vi "Fsweep_SR8XX.vi"() -> ()   [LabVIEW 2025]
panel:
  out "Array":dbl[](array[numeric])=[40.99999999999999, 50.30821597193005, 61.72967303117947, 75.74413957876105, 92.94030567161772, 114.04051146890099, 139.93108976894726, 171.6995972020422, 210.68049800813995, 258.511219387007, 317.2009330753302, 389.2149523817426, 477.57828985183363, 586.0027255944161, 719.042723886428, 882.2867474712998, 1082.5920058770212, 1328.3724985645404, 1629.9524524135916, 2000.0000000000002]
  in  "data acq time (s)":dbl=2.0
  in  "restart":bool
  in  "stop":bool
  in  "coupled device":enum16{"SRS 8XXX", "Keithley 6221"}(ring)
  in  "base delay (ms)":dbl=2000.0
  in  "test mode":bool
  out "done":u32=1
  out "delays (ms)":dbl[](array[numeric])=[4439.024390243903, 3987.7468931873063, 3619.966461664074, 3320.2341535085625, 3075.9594481357317, 2876.881370593205, 4439.024390243903, 3987.7468931873063, 3619.966461664074, 3320.2341535085625, 3075.9594481357317, 2876.881370593205, 2714.6374702370927, 4439.024390243903, 3987.7468931873063, 3619.966461664074, 3320.2341535085625, 3075.9594481357317, 2876.881370593205, 2714.6374702370927]
  in  "back to initial frequencies":bool=TRUE
  out "delay sum (min)":dbl=1.823145218207876
  in  "index offset":u16=150
  out "freq profile":dbl[][](array[numeric])=[[40.99999999999999, 171.6995972020422, 719.042723886428], [50.30821597193005, 210.68049800813995, 882.2867474712998], [61.72967303117947, 258.511219387007, 1082.5920058770212], [75.74413957876105, 317.2009330753302, 1328.3724985645404], [92.94030567161772, 389.2149523817426, 1629.9524524135916], [114.04051146890099, 477.57828985183363, 2000.0000000000002], [139.93108976894726, 586.0027255944161, 40.99999999999999], [171.6995972020422, 719.042723886428, 50.30821597193005], [210.68049800813995, 882.2867474712998, 61.72967303117947], [258.511219387007, 1082.5920058770212, 75.74413957876105], [317.2009330753302, 1328.3724985645404, 92.94030567161772], [389.2149523817426, 1629.9524524135916, 114.04051146890099], [477.57828985183363, 2000.0000000000002, 139.93108976894726], [586.0027255944161, 40.99999999999999, 171.6995972020422], [719.042723886428, 50.30821597193005, 210.68049800813995], [882.2867474712998, 61.72967303117947, 258.511219387007], [1082.5920058770212, 75.74413957876105, 317.2009330753302], [1328.3724985645404, 92.94030567161772, 389.2149523817426], [1629.9524524135916, 114.04051146890099, 477.57828985183363], [2000.0000000000002, 139.93108976894726, 586.0027255944161]]
  out "freqs":dbl[](array[numeric])=[40.99999999999999, 171.6995972020422, 719.042723886428]
  out "delay (ms)":dbl=2714.6374702370927
  out "elapsed time (min)":dbl=2.0671833333333334
  in  "sweep mode":T1(ring)=enum."log"
  in  "size":u32=200
  in  "final":dbl=2000.0
  in  "initial":dbl=41.0
  in  "Device address":refnum<visa-resource-name>[](array[refnum])=["GPIB0::1::INSTR", "GPIB0::4::INSTR", "GPIB0::7::INSTR"]
  # "Test the frequency profile and the estimated measurement time (delay sum (min)) with the 'test mode on'\nTurn the test mode off for the real measurement."
  # "Start data acquistion and frequency sweeps.\nStop the data acqusition when the sweep is done.\nRepeat when 'restart' switch is ON.\nVISA resource is reused."
  # "this delay time is added to the frequency dependent delay time"
  # "(1) For multiple lockins, the same freq profile is used but\nbut the starting frequency is offset to prevent crosstalking.\n(2) Ignored for a single lockin. \n* Check the context help"
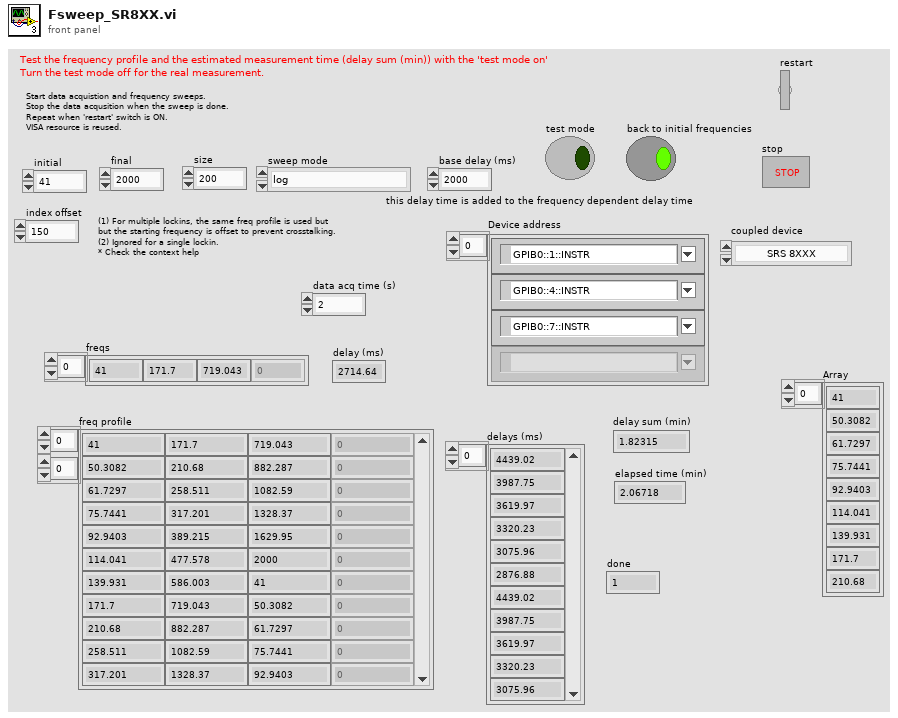
[diagram p1: front panel]
types:
  T1 = enum16{"linear", "inverse", "log", "inverse log"}
  T2 = enum32{"New", "Stop", "Trigger", "Delta Trigger", "Run", "Pause", "comments", "Started?"}
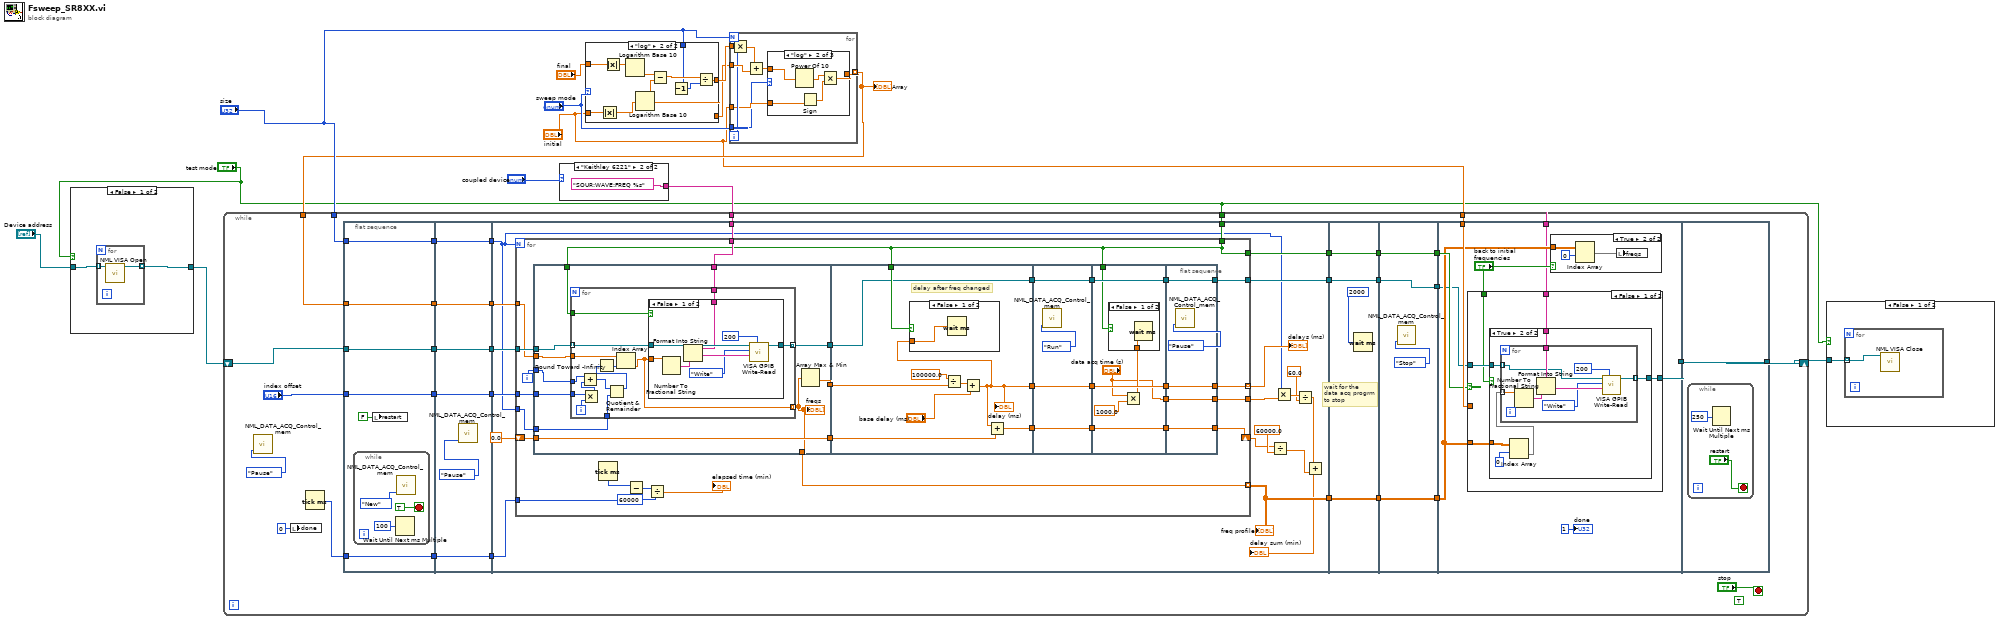
[diagram p0: block diagram]
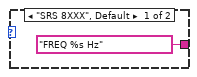
[diagram p10: hidden frame]
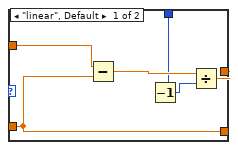
[diagram p11: hidden frame]
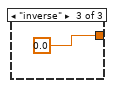
[diagram p13: hidden frame]
diagram:
  n1 = case shown="False" "test mode" {
    tunnel: [w15 w18] -> w4
    tunnel: "Device address" -> [w14 w18]
    frame False {
      n2 = for {
        tunnel: w14 -> [w17] mode=indexing
        tunnel: [w16] -> w15 mode=indexing
        n3 = call "NML VISA Open.vi"("VISA resource name"=w17) -> ("VISA resource name out"=w16:refnum<visa-resource-name>)  [unwired: 9 in, 1 out]
      }
    }
    frame True {
    }
  }
  n4 = case shown="\"Keithley 6221\"" "coupled device" {
    tunnel: ["FREQ %s Hz" ("format string") "SOUR:WAVE:FREQ %s" ("format string")] -> w5
    frame "SRS 8XXX", Default {
    }
    frame "Keithley 6221" {
    }
  }
  n5 = case shown="\"log\"" "sweep mode" {
    tunnel: "final" -> [w26 w27]
    tunnel: "initial" -> [w21 w32]
    tunnel: "size" -> [w24 w35]
    tunnel: [w23 w34] -> w13
    tunnel: [w21 w28] -> w12
    frame "linear", Default {
      n6 = Subtract(x=w26, y=w21) -> (x-y=w25:dbl)
      n7 = Decrement(x=w24) -> (x-1=w22:u32)
      n8 = Divide(x=w25, y=w22) -> (x/y=w23:dbl)
    }
    frame "log" {
      n9 = Absolute Value(x=w32) -> (abs(x)=w29:dbl)
      n10 = Absolute Value(x=w27) -> (abs(x)=w30:dbl)
      n11 = Logarithm Base 10(1:w30) -> (0:w31:dbl)
      n12 = Logarithm Base 10(1:w29) -> (0:w28:dbl)
      n13 = Subtract(x=w31, y=w28) -> (x-y=w36:dbl)
      n14 = Decrement(x=w35) -> (x-1=w33:u32)
      n15 = Divide(x=w36, y=w33) -> (x/y=w34:dbl)
    }
  }
  n16 = for {
    N: "size" -> [_]
    tunnel: w13 -> [w42]
    tunnel: [w44] -> w8 mode=indexing
    tunnel: "sweep mode" -> [w37]
    tunnel: w12 -> [w40]
    tunnel: "initial" -> [w38]
    i -> [w39]
    n17 = Multiply(x=w42, y=w39) -> (x*y=w41:dbl)
    n18 = Add(x=w41, y=w40) -> (x+y=w43:dbl)
    n19 = case shown="\"log\"" w37 {
      tunnel: [w45 w48 0.0] -> w44
      tunnel: w43 -> [w45 w50 _]
      tunnel: w38 -> [_ w47 _]
      frame "linear", Default {
      }
      frame "log" {
        n20 = Power Of 10(x=w50) -> (10^x=w49:dbl)
        n21 = Sign(1:w47) -> (0:w46:dbl)
        n22 = Multiply(x=w49, y=w46) -> (x*y=w48:dbl)
      }
      frame "inverse" {
      }
    }
  }
  "Array" <- w8
  n23 = while {
    tunnel: "size" -> [w55]
    tunnel: w8 -> [w61]
    tunnel: "initial" -> [w60]
    tunnel: w5 -> [w59]
    shift-right: [w57] -> w3
    shift-left: w4 -> [w58]
    tunnel: "test mode" -> [w53]
    stop <- "stop" stop-if-true
    (unwired) TRUE
    n24 = call "NML_DATA_ACQ_Control_mem.vi"("Enum"=T2."Pause") -> ()  [unwired: 5 in, 1 out]
    n25 = local write "done"(u32 0 ("done")) -> ()
    n26 = Tick Count (ms)() -> (millisecond timer value=w64:u32)
    n27 = flat-sequence {
      tunnel: "index offset" -> [w85]
      tunnel: w58 -> [w86]
      tunnel: w55 -> [w87]
      tunnel: w64 -> [w88]
      tunnel: w61 -> [w89]
      tunnel: [w89] -> w83
      tunnel: [w88] -> w82
      tunnel: [w87] -> w81
      tunnel: [w86] -> w80
      tunnel: [w85] -> w79
      tunnel: w83 -> [w98]
      tunnel: [w98] -> w78
      tunnel: w82 -> [w97]
      tunnel: [w97] -> w77
      tunnel: w81 -> [w96]
      tunnel: [w96] -> w76
      tunnel: w80 -> [w95]
      tunnel: [w95] -> w75
      tunnel: w79 -> [w94]
      tunnel: [w94] -> w74
      tunnel: [w117] -> w73
      tunnel: [w110] -> w72
      tunnel: w59 -> [w108]
      tunnel: [w107] -> w71
      tunnel: w78 -> [w118]
      tunnel: w77 -> [w116]
      tunnel: w76 -> [w104]
      tunnel: w75 -> [w111]
      tunnel: w74 -> [w115]
      tunnel: w53 -> [w106]
      tunnel: w73 -> [w214]
      tunnel: [w214] -> w70
      tunnel: w72 -> [w213]
      tunnel: [w213] -> w69
      tunnel: w71 -> [w212]
      tunnel: [w212] -> w68
      tunnel: w70 -> [w218]
      tunnel: [w218] -> w67
      tunnel: w69 -> [w217]
      tunnel: [w217] -> w66
      tunnel: [w216] -> w65
      tunnel: w68 -> [w216]
      tunnel: w67 -> [w225]
      tunnel: w60 -> [w226]
      tunnel: w66 -> [w222]
      tunnel: w59 -> [w221]
      tunnel: w65 -> [w219]
      tunnel: [w220] -> w54
      tunnel: [w251] -> w57
      tunnel: w54 -> [w251]
      frame #0 {
        n28 = while {
          stop <- TRUE stop-if-true
          n29 = Wait Until Next ms Multiple(millisecond multiple=u32 100) -> ()  [unwired: 1 out]
          n30 = call "NML_DATA_ACQ_Control_mem.vi"("Enum"=T2."New") -> ()  [unwired: 5 in, 1 out]
        }
        n31 = local write "restart"(FALSE ("restart")) -> ()
      }
      frame #1 {
        n32 = call "NML_DATA_ACQ_Control_mem.vi"("Enum"=T2."Pause") -> ()  [unwired: 5 in, 1 out]
      }
      frame #2 {
        n33 = for {
          N: w104 -> [_]
          tunnel: w118 -> [w135]
          tunnel: [w120] -> w117
          tunnel: w116 -> [w148]
          tunnel: w111 -> [w144]
          tunnel: w115 -> [w142]
          tunnel: w104 -> [w141]
          tunnel: [w136] -> w110 mode=indexing
          tunnel: [w119] -> w109 mode=indexing
          shift-right: [w139] -> w112
          shift-left: 0.0 -> [w137]
          tunnel: w108 -> [w134]
          tunnel: [w133] -> w107
          tunnel: w106 -> [w120]
          tunnel: [w121] -> w105
          i -> [w143]
          n34 = flat-sequence {
            tunnel: w135 -> [w158]
            tunnel: w120 -> [w160]
            tunnel: w144 -> [w159]
            tunnel: w143 -> [w157]
            tunnel: w142 -> [w156]
            tunnel: w141 -> [w155]
            tunnel: [w153] -> w140
            tunnel: [w152] -> w136
            tunnel: [w154] -> w138
            tunnel: w137 -> [w154]
            tunnel: w134 -> [w151]
            tunnel: [w150] -> w132
            tunnel: w140 -> [w191]
            tunnel: w120 -> [w189]
            tunnel: w138 -> [w186]
            tunnel: w132 -> [w184]
            tunnel: [w188] -> w131
            tunnel: [w187] -> w130
            tunnel: [w184] -> w129
            tunnel: w131 -> [w197]
            tunnel: w130 -> [w196]
            tunnel: w129 -> [w195]
            tunnel: [w197] -> w128
            tunnel: [w196] -> w127
            tunnel: [w195] -> w126
            tunnel: w128 -> [w204]
            tunnel: w127 -> [w203]
            tunnel: w126 -> [w202]
            tunnel: [w204] -> w125
            tunnel: [w203] -> w124
            tunnel: [w202] -> w123
            tunnel: ["data acq time (s)"] -> w122
            tunnel: w120 -> [w199]
            tunnel: [w208] -> w133
            tunnel: [w209] -> w139
            tunnel: [w210] -> w119
            tunnel: w125 -> [w210]
            tunnel: w124 -> [w209]
            tunnel: w123 -> [w208]
            tunnel: w122 -> [w206]
            tunnel: [w206] -> w121
            frame #0 {
              n35 = for {
                tunnel: w160 -> [w174]
                tunnel: w159 -> [w173] mode=indexing
                tunnel: w158 -> [w168]
                tunnel: w157 -> [w171]
                tunnel: w156 -> [w170]
                tunnel: [w165] -> w152 mode=indexing
                tunnel: w155 -> [w166]
                tunnel: w151 -> [w162]
                tunnel: [w161] -> w150 mode=indexing
                i -> [w172]
                n36 = Multiply(x=w170, y=w172) -> (x*y=w169:i32)
                n37 = Add(x=w171, y=w169) -> (x+y=w167:i32)
                n38 = Quotient & Remainder(x=w167, y=w166) -> (x-y*floor(x/y)=w164:u32)  [unwired: 1 out]
                n39 = Round Toward -Infinity(1:w164) -> (0:w163:u32)
                n40 = Index Array(array=w168, index=w163) -> (element=w165:dbl)
                n41 = case shown="False" w174 {
                  tunnel: w173 -> [w178 w183]
                  tunnel: w165 -> [w177 _]
                  tunnel: w162 -> [w176 _]
                  tunnel: [w175 w183] -> w161
                  frame False {
                    n42 = Number To Fractional String(number=w177) -> (F-format string=w181:string)  [unwired: 3 in]
                    n43 = Format Into String(format string=w176, w181) -> (resulting string=w182:string)  [unwired: 2 in, 1 out]
                    n44 = call "VISA GPIB Write-Read.vi"("Wait (ms)"=u32 200 ("wait (mS)"), "Command"=w182, "Action"=enum16{"Write", "Read", "Write & Read"}."Write", "VISA resource name"=w178) -> ("dup VISA Session"=w175:refnum<visa-resource-name>)  [unwired: 4 in, 3 out]
                  }
                  frame True {
                  }
                }
              }
              "freqs" <- w152
              n45 = Array Max & Min(array=w152) -> (min value=w153:dbl)  [unwired: 3 out]
            }
            frame #1 {
              # "delay after freq changed"
              n46 = Divide(x=100000.0, y=w191) -> (x/y=w192:dbl)
              n47 = Add(x=w192, y="base delay (ms)") -> (x+y=w188:dbl)
              "delay (ms)" <- w188
              n48 = case shown="False" w189 {
                tunnel: w188 -> [w193 _]
                frame False {
                  n49 = Wait (ms)(milliseconds to wait=w193) -> ()  [unwired: 1 out]
                }
                frame True {
                }
              }
              n50 = Add(x=w188, y=w186) -> (x+y=w187:dbl)
            }
            frame #2 {
              n51 = call "NML_DATA_ACQ_Control_mem.vi"("Enum"=T2."Run") -> ()  [unwired: 5 in, 1 out]
            }
            frame #3 {
              n52 = Multiply(x="data acq time (s)", y=1000.0) -> (x*y=w200:dbl)
              n53 = case shown="False" w199 {
                tunnel: w200 -> [w205 _]
                frame False {
                  n54 = Wait (ms)(milliseconds to wait=w205) -> ()  [unwired: 1 out]
                }
                frame True {
                }
              }
            }
            frame #4 {
              n55 = call "NML_DATA_ACQ_Control_mem.vi"("Enum"=T2."Pause") -> ()  [unwired: 5 in, 1 out]
            }
          }
          n56 = Tick Count (ms)() -> (millisecond timer value=w149:u32)
          n57 = Subtract(x=w149, y=w148) -> (x-y=w147:u32)
          n58 = Divide(x=w147, y=u32 60000) -> (x/y=→"elapsed time (min)":dbl)
        }
        "freq profile" <- w110
        "delays (ms)" <- w109
        n59 = Divide(x=w112, y=60000.0) -> (x/y=w100:dbl)
        n60 = Multiply(x=w104, y=w105) -> (x*y=w103:dbl)
        n61 = Divide(x=w103, y=60.0) -> (x/y=w101:dbl)
        n62 = Add(x=w101, y=w100) -> (x+y=→"delay sum (min)":dbl)
      }
      frame #3 {
        # "wait for the\ndata acq progrm\nto stop"
        n63 = Wait (ms)(milliseconds to wait=u32 2000) -> ()  [unwired: 1 out]
      }
      frame #4 {
        n64 = call "NML_DATA_ACQ_Control_mem.vi"("Enum"=T2."Stop") -> ()  [unwired: 5 in, 1 out]
      }
      frame #5 {
        n65 = case shown="False" w225 {
          tunnel: w226 -> [_ _]
          tunnel: w219 -> [w234 w250]
          tunnel: w222 -> [w233 _]
          tunnel: "back to initial frequencies" -> [w232 _]
          tunnel: w221 -> [w231 _]
          tunnel: [w230 w250] -> w220
          frame False {
            n66 = case shown="True" w232 {
              tunnel: w234 -> [w235 w241]
              tunnel: w233 -> [_ w240]
              tunnel: w231 -> [_ w237]
              tunnel: [w235 w236] -> w230
              frame False {
              }
              frame True {
                n67 = Index Array(array=w240, index (row)=0) -> (element=w238:dbl[])  [unwired: 1 in]
                n68 = for {
                  tunnel: w241 -> [w242] mode=indexing
                  tunnel: w238 -> [w245] mode=indexing
                  tunnel: w237 -> [w244]
                  tunnel: [w243] -> w236 mode=indexing
                  n69 = Number To Fractional String(number=w245) -> (F-format string=w248:string)  [unwired: 3 in]
                  n70 = Format Into String(format string=w244, w248) -> (resulting string=w249:string)  [unwired: 2 in, 1 out]
                  n71 = call "VISA GPIB Write-Read.vi"("Wait (ms)"=u32 200 ("wait (mS)"), "Command"=w249, "Action"=enum16{"Write", "Read", "Write & Read"}."Write", "VISA resource name"=w242) -> ("dup VISA Session"=w243:refnum<visa-resource-name>)  [unwired: 4 in, 3 out]
                }
              }
            }
          }
          frame True {
          }
        }
        n72 = case shown="True" "back to initial frequencies" {
          tunnel: w222 -> [_ w229]
          frame False {
          }
          frame True {
            n73 = Index Array(array=w229, index (row)=0) -> (element=w227:dbl[])  [unwired: 1 in]
            n74 = local write "freqs"(w227) -> ()
          }
        }
        "done" <- u32 1 ("done")
      }
      frame #6 {
        n75 = while {
          stop <- "restart" stop-if-true
          n76 = Wait Until Next ms Multiple(millisecond multiple=u32 250) -> ()  [unwired: 1 out]
        }
      }
    }
  }
  n77 = case shown="False" "test mode" {
    tunnel: w3 -> [w254 _]
    frame False {
      n78 = for {
        tunnel: w254 -> [w255] mode=indexing
        n79 = call "NML VISA Close.vi"("VISA resource name"=w255) -> ()  [unwired: 10 in, 1 out]
      }
    }
    frame True {
    }
  }
